vi "InitPanels.vi"(8 "error in (no error)":errorcluster, 11 "Bouncer in":refnum<class "Bouncer.lvclass">) -> (0 "error out":errorcluster, 3 "Bouncer out":refnum<class "Bouncer.lvclass">)   [LabVIEW 2019, in "RT_Game.lvlib" / "Bouncer.lvclass"]
uses:
  Bouncer.lvclass
  C:/Users/FreshBob/Dropbox/VIs/myRIO_GameConsole/RT/RT_Game/Game/Game.lvclass
  Game/Game.lvclass/Game.ctl
  BouncePanel/BouncePanel.lvclass
  C:/Users/FreshBob/Dropbox/VIs/myRIO_GameConsole/RT/RT_Game/PongPanel/PongPanel.lvclass
  C:/Users/FreshBob/Dropbox/VIs/myRIO_GameConsole/RT/RT_Game/GameObject/GameObject.lvclass
  C:/Users/FreshBob/Dropbox/VIs/myRIO_GameConsole/RT/RT_Game/RT_Sprite/RT_Sprite.lvclass
  Engine/Coordinate.ctl
  PongPanel/PongPanel.lvclass/PongPanel.ctl
  GameObject/GameObject.lvclass/GameObject.ctl
  Bouncer.lvclass/Bouncer.ctl
  PongPanel/Write StartPos.vi
  PongPanel/Write limit_y.vi
  PongPanel/Write limit_y_down.vi
  PongPanel/Write Speed.vi
  PongPanel/Write limit_x_down.vi
  PongPanel/Write limit_x_up.vi
  GameObject/Write IsActive.vi
  Game/Read Singleplayer.vi
  Engine/Engine.lvclass
  RT_Sprite/RT_Sprite.lvclass
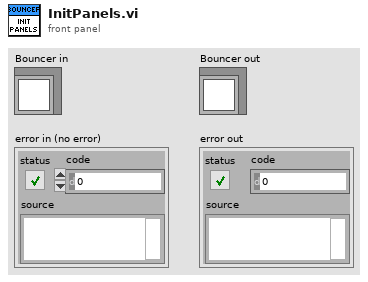
[diagram p1: front panel]
types:
  T1 = typedef "RT_Game.lvlib/Engine.lvclass/Coordinate.ctl" = cluster{"x":dbl, "y":dbl}
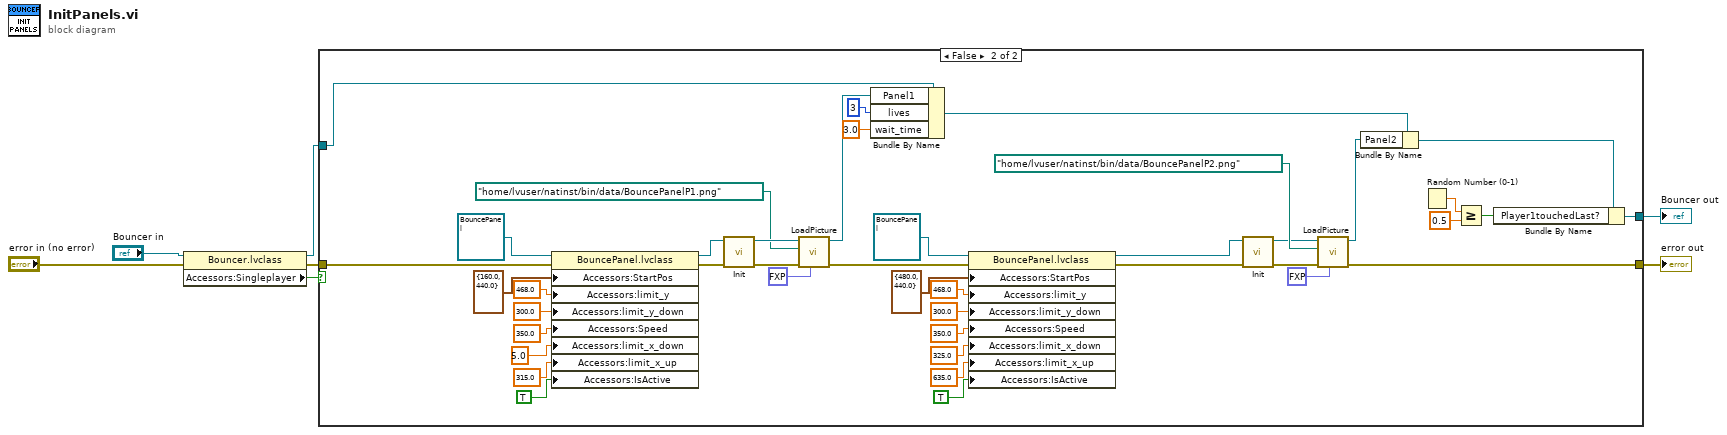
[diagram p0: block diagram]
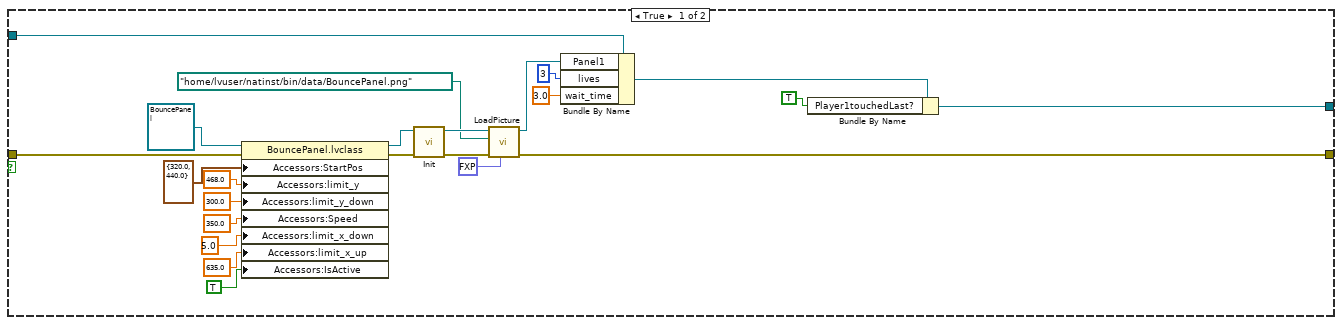
[diagram p2: hidden frame]
diagram:
  n1 = property class="Bouncer.lvclass"(reference="Bouncer in", error in="error in (no error)") -> (reference out=w4:refnum<class "Bouncer.lvclass">, error out=w2:errorcluster, "Accessors:Singleplayer"=w5:bool)
  n2 = case shown="False" w5 {
    tunnel: w2 -> [w30 w72]
    tunnel: w4 -> [w12 w32]
    tunnel: [w9 w33] -> w7
    tunnel: [w10 w37] -> w6
    frame True {
      n3 = property class="BouncePanel.lvclass"(reference=refnum<class "BouncePanel.lvclass"> refnum ("RT_Game.lvlib:BouncePanel.lvclass"), error in=w30, "Accessors:StartPos"=T1 {"x"=320.0, "y"=440.0} ("StartPos"), "Accessors:limit_y"=468.0 ("limit_y"), "Accessors:limit_y_down"=300.0 ("limit_y_down"), "Accessors:Speed"=350.0 ("Speed"), "Accessors:limit_x_down"=5.0 ("limit_x_down"), "Accessors:limit_x_up"=635.0 ("limit_x_up"), "Accessors:IsActive"=TRUE ("IsActive")) -> (reference out=w26:refnum<class "BouncePanel.lvclass">, error out=w28:errorcluster)
      n4 = call-dynamic "Init.vi"("error in (no error)"=w28, "PongPanel in"=w26) -> ("error out"=w29:errorcluster, "PongPanel out"=w19:refnum<class "BouncePanel.lvclass">)  [unwired: 8 in]
      n5 = call "LoadPicture.vi"("Transparent Color"=fxp<+,3,3> 4.0, "error in (no error)"=w29, "Picture Path"=path "/home/lvuser/natinst/bin/data/BouncePanel.png", "RT_Sprite in"=w19) -> ("error out"=w10:errorcluster, "RT_Sprite out"=w16:refnum<class "BouncePanel.lvclass">)  [unwired: 6 in]
      n6 = Bundle By Name(cluster=w12, "Panel1"=w16, "lives"=i16 3, "wait_time"=3.0) -> (w11:refnum<class "Bouncer.lvclass">)
      n7 = Bundle By Name(cluster=w11, "Player1touchedLast?"=TRUE) -> (w9:refnum<class "Bouncer.lvclass">)
    }
    frame False {
      n8 = property class="BouncePanel.lvclass"(reference=refnum<class "BouncePanel.lvclass"> refnum ("RT_Game.lvlib:BouncePanel.lvclass"), error in=w72, "Accessors:StartPos"=T1 {"x"=160.0, "y"=440.0} ("StartPos"), "Accessors:limit_y"=468.0 ("limit_y"), "Accessors:limit_y_down"=300.0 ("limit_y_down"), "Accessors:Speed"=350.0 ("Speed"), "Accessors:limit_x_down"=5.0 ("limit_x_down"), "Accessors:limit_x_up"=315.0 ("limit_x_up"), "Accessors:IsActive"=TRUE ("IsActive")) -> (reference out=w68:refnum<class "BouncePanel.lvclass">, error out=w70:errorcluster)
      n9 = call-dynamic "Init.vi"("error in (no error)"=w70, "PongPanel in"=w68) -> ("error out"=w71:errorcluster, "PongPanel out"=w61:refnum<class "BouncePanel.lvclass">)  [unwired: 8 in]
      n10 = call "LoadPicture.vi"("Transparent Color"=fxp<+,3,3> 4.0, "error in (no error)"=w71, "Picture Path"=path "/home/lvuser/natinst/bin/data/BouncePanelP1.png", "RT_Sprite in"=w61) -> ("error out"=w39:errorcluster, "RT_Sprite out"=w58:refnum<class "BouncePanel.lvclass">)  [unwired: 6 in]
      n11 = Bundle By Name(cluster=w32, "Panel1"=w58, "lives"=i16 3, "wait_time"=3.0) -> (w31:refnum<class "Bouncer.lvclass">)
      n12 = property class="BouncePanel.lvclass"(reference=refnum<class "BouncePanel.lvclass"> refnum ("RT_Game.lvlib:BouncePanel.lvclass"), error in=w39, "Accessors:StartPos"=T1 {"x"=480.0, "y"=440.0} ("StartPos"), "Accessors:limit_y"=468.0 ("limit_y"), "Accessors:limit_y_down"=300.0 ("limit_y_down"), "Accessors:Speed"=350.0 ("Speed"), "Accessors:limit_x_down"=325.0 ("limit_x_down"), "Accessors:limit_x_up"=635.0 ("limit_x_up"), "Accessors:IsActive"=TRUE ("IsActive")) -> (reference out=w43:refnum<class "BouncePanel.lvclass">, error out=w41:errorcluster)
      n13 = call-dynamic "Init.vi"("error in (no error)"=w41, "PongPanel in"=w43) -> ("error out"=w40:errorcluster, "PongPanel out"=w50:refnum<class "BouncePanel.lvclass">)  [unwired: 8 in]
      n14 = call "LoadPicture.vi"("Transparent Color"=fxp<+,3,3> 4.0, "error in (no error)"=w40, "Picture Path"=path "/home/lvuser/natinst/bin/data/BouncePanelP2.png", "RT_Sprite in"=w50) -> ("error out"=w37:errorcluster, "RT_Sprite out"=w53:refnum<class "BouncePanel.lvclass">)  [unwired: 6 in]
      n15 = Bundle By Name(cluster=w31, "Panel2"=w53) -> (w38:refnum<class "Bouncer.lvclass">)
      n16 = Random Number (0-1)() -> (number: 0 to 1=w36:dbl)
      n17 = Greater Or Equal?(x=w36, y=0.5) -> (x >= y?=w34:bool)
      n18 = Bundle By Name(cluster=w38, "Player1touchedLast?"=w34) -> (w33:refnum<class "Bouncer.lvclass">)
    }
  }
  "Bouncer out" <- w7
  "error out" <- w6
